vi "ATM Message Handler.vi"(8 "error in (no error)":errorcluster, 10 "Parameters":string[](array[string]), 11 "Message Name":string) -> (0 "error out":errorcluster, 3 "Message":string)   [LabVIEW 2011]
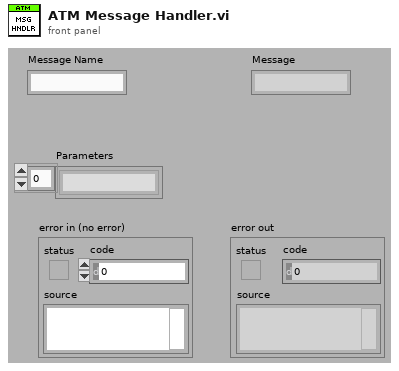
[diagram p1: front panel]
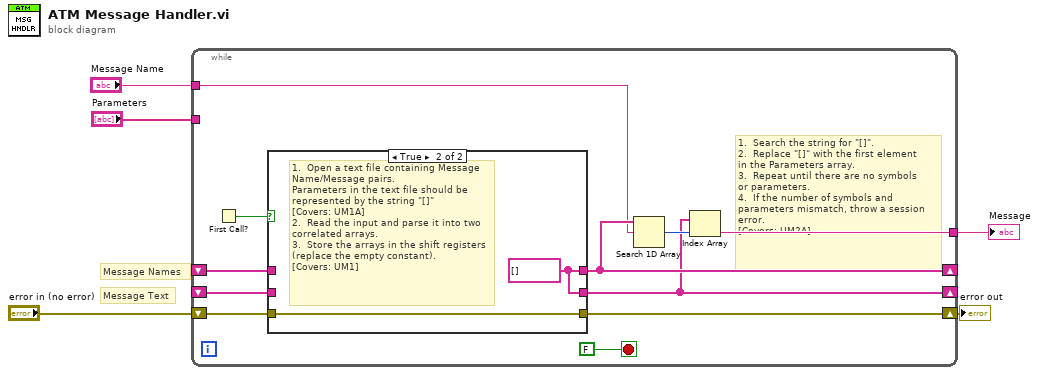
[diagram p0: block diagram]
diagram:
  # "Message Text"
  # "Message Names"
  n1 = while {
    shift-right: [w14] -> w4
    shift-left: "error in (no error)" -> [w15]
    shift-right: [w10] -> _
    shift-left: _ -> [w12]
    shift-right: [w7] -> _
    shift-left: _ -> [w11]
    tunnel: "Message Name" -> [w9]
    tunnel: "Parameters" -> [_]
    tunnel: [w6] -> w1
    stop <- FALSE stop-if-true
    # "1.  Search the string for \"[]\".\n2.  Replace \"[]\" with the first element\nin the Parameters array.\n3.  Repeat until there are no symbols\nor parameters.\n4.  If the number of symbols and\nparameters mismatch, throw a session\nerror.\n[Covers: UM2A]"
    n2 = First Call?() -> (First Call?: T/F=w16:bool)
    n3 = case shown="True" w16 {
      tunnel: w15 -> [w17 w21]
      tunnel: [w17 w21] -> w14
      tunnel: [w19 w20] -> w10
      tunnel: [w18 w20] -> w7
      tunnel: w12 -> [w19 _]
      tunnel: w11 -> [w18 _]
      frame False {
      }
      frame True {
        w20 = string[] [] ("Parameters")
        # "1.  Open a text file containing Message Name/Message pairs.\nParameters in the text file should be represented by the string \"[]\"\n[Covers: UM1A]\n2.  Read the input and parse it into two correlated arrays.\n3.  Store the arrays in the shift registers (replace the empty constant).\n[Covers: UM1]"
      }
    }
    n4 = Search 1D Array(1D array=w10, element=w9) -> (index of element=w8:i32)  [unwired: 1 in]
    n5 = Index Array(array=w7, index=w8) -> (element=w6:string)
  }
  "Message" <- w1
  "error out" <- w4
